vi "Initialise RT system.vi"(9 "CompressorRigV2":T1, 11 "config data out":T18={"Message"={"Parameters"={"FPGA Ref"=refnum, "configID"=0, "activeChannels"=[]}, "Variables"={"RT Status"={"Comms loop"=FALSE, "scheduler loop"=FALSE, "data process loop"=FALSE, "FIFO loop"=FALSE, "Command Stream"=FALSE, "Error Stream"=FALSE, "FPGA FIFO"=FALSE, "Data Stream"=FALSE}, "watchdog"=timestamp(0 s since 1904-01-01), "limitsEnabled"=FALSE, "Interlocks"={"gearboxOil"=FALSE, "bearingOil"=FALSE, "gearboxAir"=FALSE}}}, "FIFO"={"Params"={"FPGA ref"=refnum, "Total Channels"=0}, "Variables"={"FIFO wait counter"=0, "FIFO read trigger"=0}}, "Comms data"={"Parameters"={"error writer name"="", "command reader name"="", "error buffer size"=0, "command buffer size"=0, "scanivalveIP"="", "scanivalvePeriod"=0}, "Variables"={"listen schedule"=0, "incident buffer"=[], "command stream"="", "error stream"="", "waiting for command stream connect"=FALSE, "waiting for error stream connect"=FALSE, "scanivalve connection"=refnum, "scanivalveScheduleID"=0, "activeScanivalvePorts"=[], "channelCount"=0}, "scanivalveConfig"={"listS"={"period"=0, "ADtrig"=FALSE, "ScanTrig"=FALSE, "page"=0, "qpkts"=0}, "listC"={"ZC"=FALSE, "unitScan"="", "CvtUnit"=0.0, "bin"=FALSE, "EU"=FALSE}, "listSG"={"Avg1"=0, "FPS1"=0, "SGEnable1"=FALSE}, "activeChannels"={"Chan1"={"101"=FALSE, "102"=FALSE, "103"=FALSE, "104"=FALSE, "109"=FALSE, "110"=FALSE, "111"=FALSE, "112"=FALSE, "201"=FALSE, "202"=FALSE, "203"=FALSE, "204"=FALSE, "209"=FALSE, "210"=FALSE, "211"=FALSE, "212"=FALSE, "301"=FALSE, "302"=FALSE, "303"=FALSE, "304"=FALSE, "309"=FALSE, "310"=FALSE, "311"=FALSE, "312"=FALSE, "401"=FALSE, "402"=FALSE, "403"=FALSE, "404"=FALSE, "409"=FALSE, "410"=FALSE, "411"=FALSE, "412"=FALSE}}}}, "Data processor"={"Parameters"={"FPGA Ref"=refnum, "data stream"={"data writer name"="error writer", "NS write buffer size"=16, "NS Buffer length"=0}, "FIFO Depth"=0, "Channel controls"={"FIFO channel count"=0, "active indices"=[], "active channels"=0, "channelScaling"=[], "scanivalveCount"=0, "channels"=[]}, "safetyChannels"={"oilP"=0, "airP"=0, "water"=0, "channelLimits"=[]}, "speedChannel"=0, "maxSpeedLimit"=0.0, "Torque"={"fixedOffset"=0.0, "filter"=FALSE, "fallingEdge"=FALSE, "swapEncoders"=FALSE}}, "Variables"={"Intermediary buffer"=[], "buffer position"=0, "write loop counter"=0, "NS write trigger"=0, "NS Connection status"=FALSE, "waiting for NS"=FALSE, "labAmbient"={"pressure"=0.0, "temperature"=0.0}, "scanivalvePorts"=[], "scanivalvePressures"=[], "data stream"="", "activeChannelLimitIndex"=[], "runningSpeedLimit"=0.0, "speedChannelIndex"=0, "Interlocks"={"gearboxOil"=FALSE, "bearingOil"=FALSE, "gearboxAir"=FALSE}, "interlockChannels"={"gearboxOil"=0, "bearingOil"=0, "air"=0}, "limitStates"=[]}}}) -> (1 "config data":T18={"Message"={"Parameters"={"FPGA Ref"=refnum, "configID"=0, "activeChannels"=[]}, "Variables"={"RT Status"={"Comms loop"=FALSE, "scheduler loop"=FALSE, "data process loop"=FALSE, "FIFO loop"=FALSE, "Command Stream"=FALSE, "Error Stream"=FALSE, "FPGA FIFO"=FALSE, "Data Stream"=FALSE}, "watchdog"=timestamp(0 s since 1904-01-01), "limitsEnabled"=FALSE, "Interlocks"={"gearboxOil"=FALSE, "bearingOil"=FALSE, "gearboxAir"=FALSE}}}, "FIFO"={"Params"={"FPGA ref"=refnum, "Total Channels"=0}, "Variables"={"FIFO wait counter"=0, "FIFO read trigger"=0}}, "Comms data"={"Parameters"={"error writer name"="", "command reader name"="", "error buffer size"=0, "command buffer size"=0, "scanivalveIP"="", "scanivalvePeriod"=0}, "Variables"={"listen schedule"=0, "incident buffer"=[], "command stream"="", "error stream"="", "waiting for command stream connect"=FALSE, "waiting for error stream connect"=FALSE, "scanivalve connection"=refnum, "scanivalveScheduleID"=0, "activeScanivalvePorts"=[], "channelCount"=0}, "scanivalveConfig"={"listS"={"period"=0, "ADtrig"=FALSE, "ScanTrig"=FALSE, "page"=0, "qpkts"=0}, "listC"={"ZC"=FALSE, "unitScan"="", "CvtUnit"=0.0, "bin"=FALSE, "EU"=FALSE}, "listSG"={"Avg1"=0, "FPS1"=0, "SGEnable1"=FALSE}, "activeChannels"={"Chan1"={"101"=FALSE, "102"=FALSE, "103"=FALSE, "104"=FALSE, "109"=FALSE, "110"=FALSE, "111"=FALSE, "112"=FALSE, "201"=FALSE, "202"=FALSE, "203"=FALSE, "204"=FALSE, "209"=FALSE, "210"=FALSE, "211"=FALSE, "212"=FALSE, "301"=FALSE, "302"=FALSE, "303"=FALSE, "304"=FALSE, "309"=FALSE, "310"=FALSE, "311"=FALSE, "312"=FALSE, "401"=FALSE, "402"=FALSE, "403"=FALSE, "404"=FALSE, "409"=FALSE, "410"=FALSE, "411"=FALSE, "412"=FALSE}}}}, "Data processor"={"Parameters"={"FPGA Ref"=refnum, "data stream"={"data writer name"="error writer", "NS write buffer size"=16, "NS Buffer length"=0}, "FIFO Depth"=0, "Channel controls"={"FIFO channel count"=0, "active indices"=[], "active channels"=0, "channelScaling"=[], "scanivalveCount"=0, "channels"=[]}, "safetyChannels"={"oilP"=0, "airP"=0, "water"=0, "channelLimits"=[]}, "speedChannel"=0, "maxSpeedLimit"=0.0, "Torque"={"fixedOffset"=0.0, "filter"=FALSE, "fallingEdge"=FALSE, "swapEncoders"=FALSE}}, "Variables"={"Intermediary buffer"=[], "buffer position"=0, "write loop counter"=0, "NS write trigger"=0, "NS Connection status"=FALSE, "waiting for NS"=FALSE, "labAmbient"={"pressure"=0.0, "temperature"=0.0}, "scanivalvePorts"=[], "scanivalvePressures"=[], "data stream"="", "activeChannelLimitIndex"=[], "runningSpeedLimit"=0.0, "speedChannelIndex"=0, "Interlocks"={"gearboxOil"=FALSE, "bearingOil"=FALSE, "gearboxAir"=FALSE}, "interlockChannels"={"gearboxOil"=0, "bearingOil"=0, "air"=0}, "limitStates"=[]}}}, 3 "Queues":T19)   [LabVIEW 2018]
doc: "Create the Queues required for the Compressor Rig RT application:\n\nMessage queue (string + variant)\nAnalogue data (double array)\nTorque data (double array)\n\nAfter initialisation an 'init' message is written to the RT Message queue"
uses:
  Type Defs/Queues cluster.ctl
  ICL-LabVIEW_General/Message Scheduler/message scheduler.lvclass
  Type Defs/Message loop data.ctl
  Type Defs/FPGA reference.ctl
  Type Defs/RT Status.ctl
  Type Defs/Analogue loop data.ctl
  Communications loop/comms data.ctl
  Type Defs/generic incident.ctl
  ICL-LabVIEW_General/Scanivalve API project/full interface/polymorphic/scanivalveConfig.ctl
  ICL-LabVIEW_General/Scanivalve API project/full interface/listS.ctl
  ICL-LabVIEW_General/Scanivalve API project/full interface/listC.ctl
  ICL-LabVIEW_General/Scanivalve API project/full interface/listSG.ctl
  ICL-LabVIEW_General/Scanivalve API project/full interface/chan1.ctl
  Type Defs/Data processing loop data.ctl
  PC/type defs/channelControl.ctl
  Type Defs/channelScalingTypes.ctl
  Type Defs/scalingMethods.ctl
  ICL-LabVIEW_General/data channels/parent class/Data Channel.lvclass
  PC/type defs/channelLimitControl.ctl
  PC/type defs/limitActions.ctl
  Type Defs/channelConfigFilePath.ctl
  ICL-LabVIEW_General/data channels/data channels.lvlib
  ICL-LabVIEW_General/Scanivalve API project/Scanivalve API.lvlib
panel:
  out "activeChannelCount":u16
  out "scanivalve":i32
  out "FIFO channels":u16
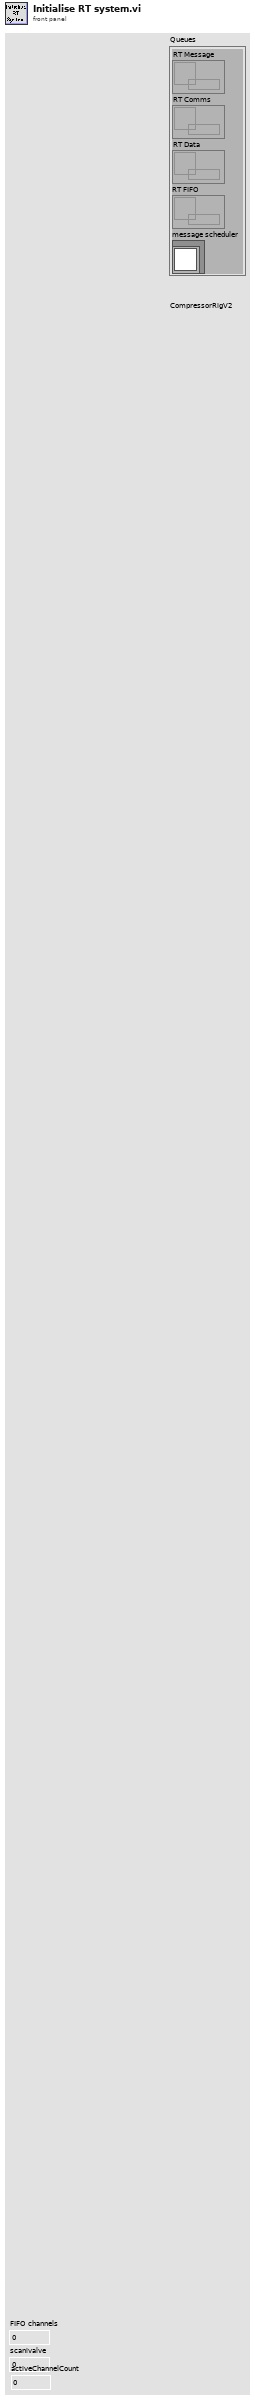
[diagram p1: front panel]
types:
  T1 = typedef "FPGA reference.ctl" = refnum<k20>
  T2 = typedef "Message loop data.ctl" = cluster{"Parameters":cluster{"FPGA Ref":T1, "configID":u32, "activeChannels":cluster{"index":u16, "name":string}[]}, "Variables":cluster{"RT Status":T3, "watchdog":timestamp, "limitsEnabled":bool, "Interlocks":cluster{"gearboxOil":bool, "bearingOil":bool, "gearboxAir":bool}}}
  T3 = typedef "RT Status.ctl" = cluster{"Comms loop":bool, "scheduler loop":bool, "data process loop":bool, "FIFO loop":bool, "Command Stream":bool, "Error Stream":bool, "FPGA FIFO":bool, "Data Stream":bool}
  T4 = typedef "Analogue loop data.ctl" = cluster{"Params":cluster{"FPGA ref":T1, "Total Channels":u32}, "Variables":cluster{"FIFO wait counter":u16, "FIFO read trigger":u32}}
  T5 = typedef "comms data.ctl" = cluster{"Parameters":cluster{"error writer name":string, "command reader name":string, "error buffer size":i32, "command buffer size":i32, "scanivalveIP":string, "scanivalvePeriod":u16}, "Variables":cluster{"listen schedule":u32, "incident buffer":T6[], "command stream":refnum<k21>, "error stream":refnum<k21>, "waiting for command stream connect":bool, "waiting for error stream connect":bool, "scanivalve connection":refnum<k5>, "scanivalveScheduleID":u32, "activeScanivalvePorts":i32[], "channelCount":i16}, "scanivalveConfig":T7}
  T6 = typedef "generic incident.ctl" = cluster{"timestamp":timestamp, "type":string, "Variant":variant}
  T7 = typedef "Scanivalve API.lvlib/scanivalveConfig.ctl" = cluster{"listS":T8, "listC":T9, "listSG":T10, "activeChannels":T11}
  T8 = typedef "Scanivalve API.lvlib/listS.ctl" = cluster{"period":u16, "ADtrig":bool, "ScanTrig":bool, "page":u16, "qpkts":u16}
  T9 = typedef "Scanivalve API.lvlib/listC.ctl" = cluster{"ZC":bool, "unitScan":string, "CvtUnit":dbl, "bin":bool, "EU":bool}
  T10 = typedef "Scanivalve API.lvlib/listSG.ctl" = cluster{"Avg1":u16, "FPS1":u16, "SGEnable1":bool}
  T11 = typedef "Scanivalve API.lvlib/chan1.ctl" = cluster{"Chan1":cluster{"101":bool, "102":bool, "103":bool, "104":bool, "109":bool, "110":bool, "111":bool, "112":bool, "201":bool, "202":bool, "203":bool, "204":bool, "209":bool, "210":bool, "211":bool, "212":bool, "301":bool, "302":bool, "303":bool, "304":bool, "309":bool, "310":bool, "311":bool, "312":bool, "401":bool, "402":bool, "403":bool, "404":bool, "409":bool, "410":bool, "411":bool, "412":bool}}
  T12 = typedef "Data processing loop data.ctl" = cluster{"Parameters":cluster{"FPGA Ref":T1, "data stream":cluster{"data writer name":string, "NS write buffer size":i32, "NS Buffer length":u32}, "FIFO Depth":u32, "Channel controls":cluster{"FIFO channel count":i32, "active indices":i16[], "active channels":i32, "channelScaling":T13[], "scanivalveCount":i32, "channels":refnum<class "Data Channel.lvclass">[]}, "safetyChannels":cluster{"oilP":u16, "airP":u16, "water":u16, "channelLimits":T16[]}, "speedChannel":i32, "maxSpeedLimit":dbl, "Torque":cluster{"fixedOffset":dbl, "filter":bool, "fallingEdge":bool, "swapEncoders":bool}}, "Variables":cluster{"Intermediary buffer":dbl[][], "buffer position":u32, "write loop counter":u16, "NS write trigger":u32, "NS Connection status":bool, "waiting for NS":bool, "labAmbient":cluster{"pressure":dbl, "temperature":dbl}, "scanivalvePorts":u16[], "scanivalvePressures":dbl[], "data stream":refnum<k21>, "activeChannelLimitIndex":u16[], "runningSpeedLimit":dbl, "speedChannelIndex":i32, "Interlocks":cluster{"gearboxOil":bool, "bearingOil":bool, "gearboxAir":bool}, "interlockChannels":cluster{"gearboxOil":i32, "bearingOil":i32, "air":i32}, "limitStates":cluster{"warn":bool, "alarm":bool}[]}}
  T13 = typedef "channelControl.ctl" = cluster{"index":u16, "active":bool, "channelType":T14, "module":u16, "terminal":u16, "channelName":string, "scalingMethod":T15, "scalingParameters":dbl[], "scaledUnits":string, "tempOffset":dbl}
  T14 = typedef "channelScalingTypes.ctl" = enum16{"calculation", "measurement", "scanivalve", "output", "digital"}
  T15 = typedef "scalingMethods.ctl" = enum16{"none", "linear", "thermocouple", "polynomial", "encoder", "RTD"}
  T16 = typedef "channelLimitControl.ctl" = cluster{"channelID":u16, "Enabled":bool, "warnValue":dbl, "limitValue":dbl, "Invert":bool, "limitAction":T17}
  T17 = typedef "limitActions.ctl" = enum16{"stop", "shutdown", "ignore"}
  T18 = cluster{"Message":T2, "FIFO":T4, "Comms data":T5, "Data processor":T12}
  T19 = typedef "Queues cluster.ctl" = cluster{"RT Message":refnum<queue>, "RT Comms":refnum<queue>, "RT Data":refnum<queue>, "RT FIFO":refnum<queue>, "message scheduler":refnum<class "message scheduler.lvclass">}
  T20 = typedef "channelConfigFilePath.ctl" = path
  T21 = cluster{"total":cluster{"channels":u16, "FIFO":u16, "Scanivalve":u16, "Remote":u16, "Calculated":u16}, "active":cluster{"channels":u16, "FIFO":u16, "Scanivalve":u16, "Remote":u16, "Calculated":u16}}
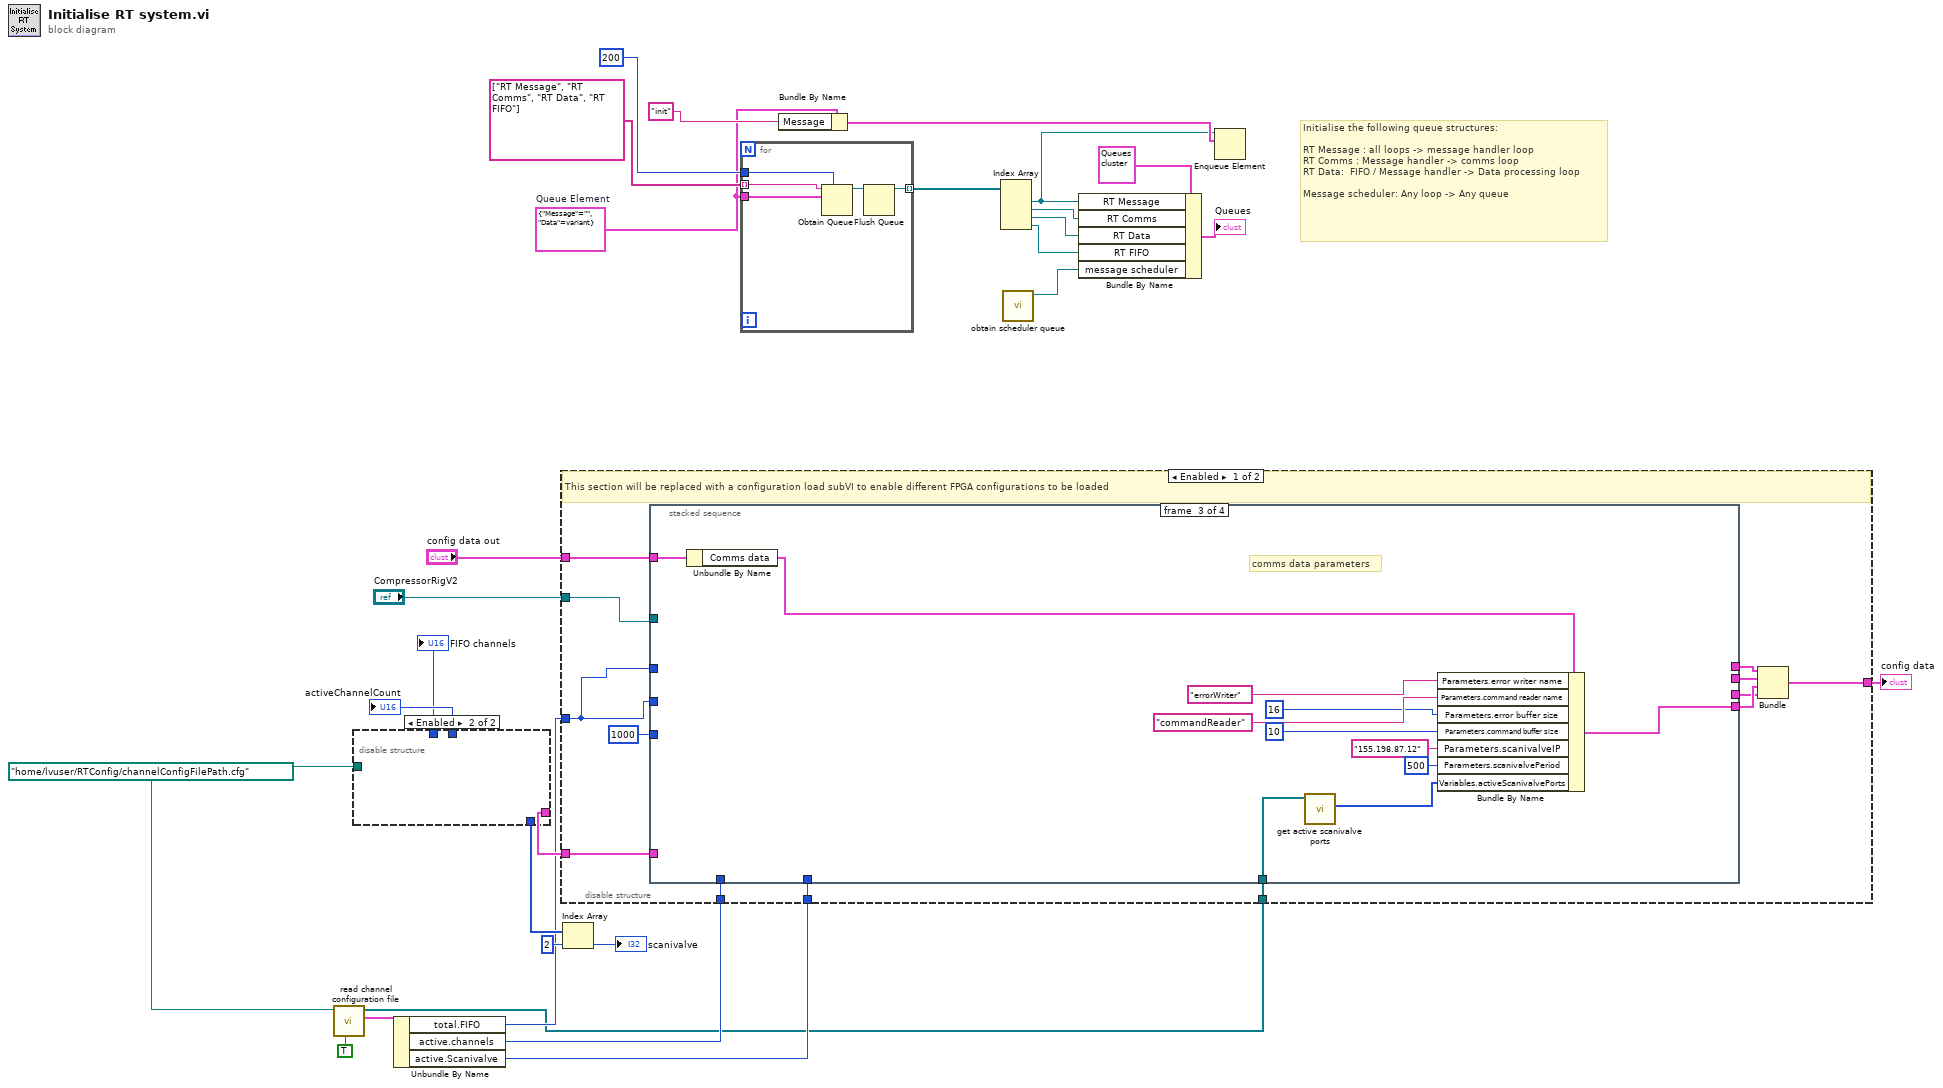
[diagram p0: block diagram]
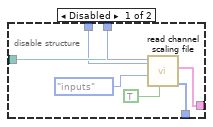
[diagram p2: hidden frame]
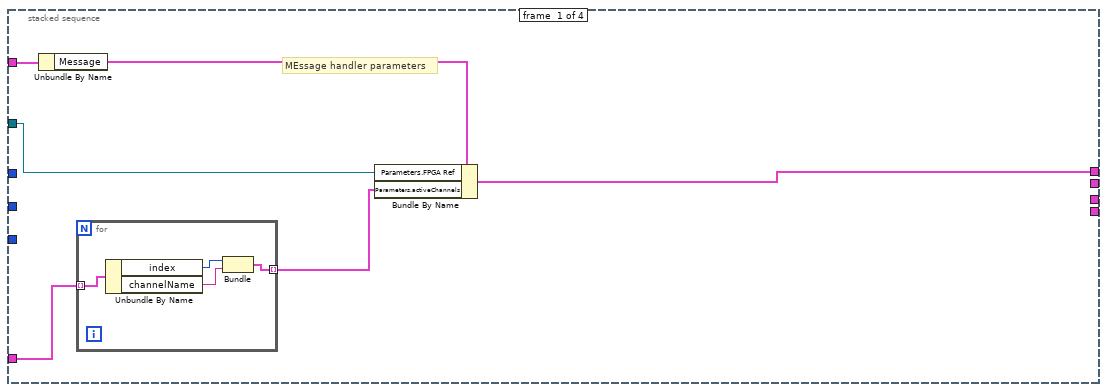
[diagram p3: hidden frame]
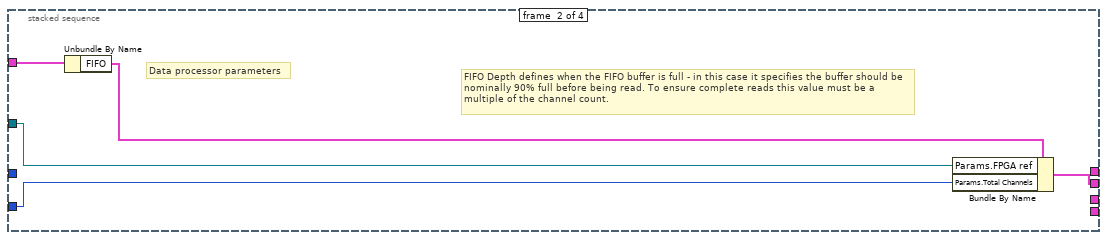
[diagram p4: hidden frame]
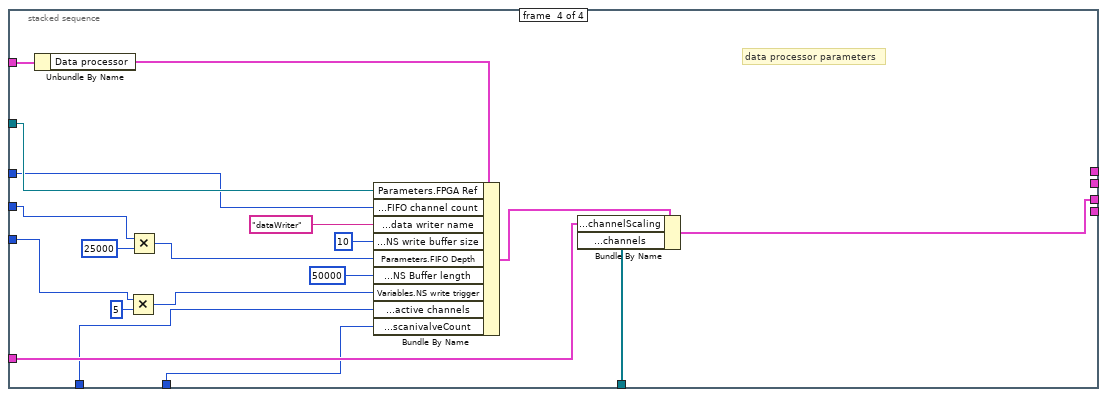
[diagram p5: hidden frame]
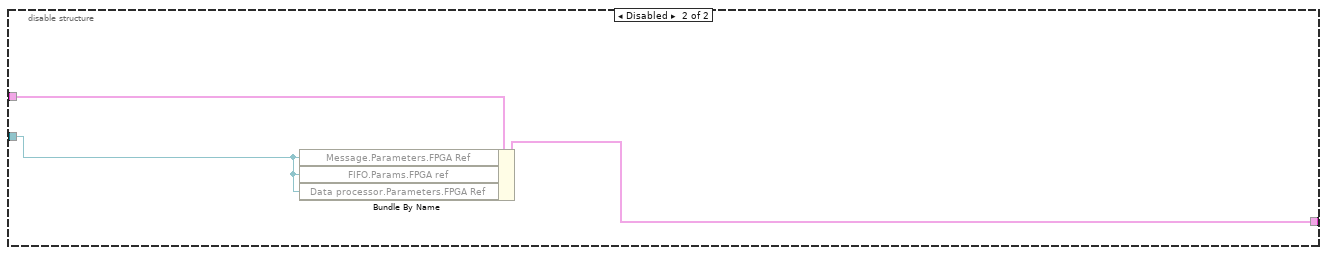
[diagram p6: hidden frame]
diagram:
  w9 = T20 path "/home/lvuser/RTConfig/channelConfigFilePath.cfg" ("channelConfigFilePath")
  w24 = cluster{"Message":string, "Data":variant} {"Message"="", "Data"=variant}  # Queue Element
  # "Initialise the following queue structures:\n\nRT Message : all loops -> message handler loop\nRT Comms : Message handler -> comms loop\nRT Data:  FIFO / Message handler -> Data processing loop\n\nMessage scheduler: Any loop -> Any queue"
  n1 = call "read channel configuration file.vi"("Hide inactive (F)"=TRUE, "config file"=w9) -> ("counts"=w5:T21, "channelsArray"=w1:refnum<class "Data Channel.lvclass">[])  [unwired: 7 in, 1 out]
  n2 = disable-structure shown="Enabled" {
    disable-tunnel: [w36 _] -> w18
    disable-tunnel: [w35 _] -> w17
    disable-tunnel: [w32 _] -> w12
    disable-tunnel: w9 -> [w31 _]
    disable-tunnel: [w30 _] -> w7
    frame Disabled {
      n3 = call "read channel scaling file.vi"("suppress inactive? (F)"=TRUE, "mode (all)"=enum16{"all", "inputs", "outputs", "digital"}."inputs", "file path"=w31) -> ("channelTypeCount"=w32:i32[], "channelConfig"=w36:T13[], "activeChannelCount"=w35:u16, "FIFO channels"=w30:u16)  [unwired: 4 in, 1 out]
    }
    frame Enabled {
    }
  }
  "FIFO channels" <- w7
  "activeChannelCount" <- w17
  n4 = Unbundle By Name(w5) -> ("total.FIFO"=w4:u16, "active.channels"=w3:u16, "active.Scanivalve"=w2:u16)
  n5 = disable-structure shown="Enabled" {
    disable-tunnel: [w44 w97] -> w14
    disable-tunnel: "CompressorRigV2" -> [w43 w96]
    disable-tunnel: w18 -> [w42 _]
    disable-tunnel: w4 -> [w41 _]
    disable-tunnel: "config data out" -> [w40 w95]
    disable-tunnel: w2 -> [w39 _]
    disable-tunnel: w1 -> [w38 _]
    disable-tunnel: w3 -> [w37 _]
    frame Enabled {
      # "This section will be replaced with a configuration load subVI to enable different FPGA configurations to be loaded"
      n6 = stacked-sequence {
        tunnel: [w55 _ _ _] -> w49
        tunnel: [_ w64 _ _] -> w48
        tunnel: w43 -> [w54 w63 _ w94]
        tunnel: [_ _ w75 _] -> w47
        tunnel: [_ _ _ w84] -> w46
        tunnel: w41 -> [_ w62 _ w89]
        tunnel: u32 1000 ("y") -> [_ _ _ w87]
        tunnel: w42 -> [w51 _ _ w83]
        tunnel: w41 -> [_ _ _ w82]
        tunnel: w40 -> [w53 w61 w68 w81]
        tunnel: w39 -> [_ _ _ w79]
        tunnel: w38 -> [_ _ w66 w77]
        tunnel: w37 -> [_ _ _ w76]
        frame #0 {
          # "MEssage handler parameters"
          n7 = Unbundle By Name(w53) -> ("Message"=w52:T2)
          n8 = for {
            tunnel: w51 -> [w59] mode=indexing
            tunnel: [w56] -> w50 mode=indexing
            n9 = Unbundle By Name(w59) -> ("index"=w58:u16, "channelName"=w57:string)
            n10 = Bundle("index"=w58, "channelName"=w57) -> (w56:cluster{"index":u16, "channelName":string})  [unwired: 1 in]
          }
          n11 = Bundle By Name(cluster=w52, "Parameters.FPGA Ref"=w54, "Parameters.activeChannels"=w50) -> (w55:T2)
        }
        frame #1 {
          # "Data processor parameters"
          # "FIFO Depth defines when the FIFO buffer is full - in this case it specifies the buffer should be nominally 90% full before being read. To ensure complete reads this value must be a multiple of the channel count."
          n12 = Unbundle By Name(w61) -> ("FIFO"=w60:T4)
          n13 = Bundle By Name(cluster=w60, "Params.FPGA ref"=w63, "Params.Total Channels"=w62) -> (w64:T4)
        }
        frame #2 {
          # "comms data parameters"
          n14 = Unbundle By Name(w68) -> ("Comms data"=w67:T5)
          n15 = call "get active scanivalve ports.vi"("channels"=w66) -> ("activeScanivalvePorts"=w65:i32[])  [unwired: 10 in]
          n16 = Bundle By Name(cluster=w67, "Parameters.error writer name"="errorWriter", "Parameters.command reader name"="commandReader", "Parameters.error buffer size"=16, "Parameters.command buffer size"=10, "Parameters.scanivalveIP"="155.198.87.12", "Parameters.scanivalvePeriod"=u16 500, "Variables.activeScanivalvePorts"=w65) -> (w75:T5)
        }
        frame #3 {
          # "data processor parameters"
          n17 = Unbundle By Name(w81) -> ("Data processor"=w80:T12)
          n18 = Multiply(x=w87, y=u32 5) -> (x*y=w90:u32)
          n19 = Multiply(x=w89, y=u32 25000) -> (x*y=w88:u32)
          n20 = Bundle By Name(cluster=w80, "Parameters.FPGA Ref"=w94, "Parameters.Channel controls.FIFO channel count"=w82, "Parameters.data stream.data writer name"="dataWriter" ("Parameters.Data stream.data writer name"), "Parameters.data stream.NS write buffer size"=10 ("Parameters.Data stream.data buffer size"), "Parameters.FIFO Depth"=w88, "Parameters.data stream.NS Buffer length"=u32 50000, "Variables.NS write trigger"=w90, "Parameters.Channel controls.active channels"=w76, "Parameters.Channel controls.scanivalveCount"=w79) -> (w85:T12)
          n21 = Bundle By Name(cluster=w85, "Parameters.Channel controls.channelScaling"=w83, "Parameters.Channel controls.channels"=w77) -> (w84:T12)
        }
      }
      n22 = Bundle("Message"=w49, "FIFO"=w48, "Comms data"=w47, "Data processor"=w46) -> (w44:T18)  [unwired: 1 in]
    }
    frame Disabled {
      n23 = Bundle By Name(cluster=w95, "Message.Parameters.FPGA Ref"=w96, "FIFO.Params.FPGA ref"=w96, "Data processor.Parameters.FPGA Ref"=w96) -> (w97:T18)
    }
  }
  "config data" <- w14
  n24 = Index Array(array=w12, index=2) -> (element=→"scanivalve":i32)
  n25 = for {
    tunnel: string[] ["RT Message", "RT Comms", "RT Data", "RT FIFO"] ("name (unnamed)") -> [w102] mode=indexing
    tunnel: 200 ("max queue size (-1, unlimited)") -> [w101]
    tunnel: [w98] -> w25 mode=indexing
    tunnel: w24 -> [w100]
    n26 = Obtain Queue(max queue size (-1, unlimited)=w101, name (unnamed)=w102, element data type=w100) -> (queue out=w99:refnum<queue>)  [unwired: 2 in, 2 out]
    n27 = Flush Queue(queue=w99) -> (queue out=w98:refnum<queue>)  [unwired: 1 in, 2 out]
  }
  n28 = Bundle By Name(cluster=w24, "Message"="init") -> (w26:cluster{"Message":string, "Data":variant})
  n29 = Index Array(array=w25) -> (element #1=w15:refnum<queue>, element #2=w21:refnum<queue>, element #3=w19:refnum<queue>, element #4=w10:refnum<queue>)  [unwired: 4 in]
  n30 = call "obtain scheduler queue.vi"() -> ("message scheduler out"=w20:refnum<class "message scheduler.lvclass">)  [unwired: 10 in, 1 out]
  n31 = Bundle By Name(cluster=T19 {"RT Message"=refnum, "RT Comms"=refnum, "RT Data"=refnum, "RT FIFO"=refnum, "message scheduler"=refnum} ("RT Queues"), "RT Message"=w15, "RT Comms"=w21, "RT Data"=w19, "RT FIFO"=w10, "message scheduler"=w20) -> (→"Queues":T19)
  n32 = Enqueue Element(queue=w15, element=w26) -> ()  [unwired: 2 in, 3 out]
